vi "KM_appendline --readfreq.vi"(1 "freq":dbl format="%#_13g", 5 "append to file? (new file:F)":bool=TRUE, 7 "Save frequency scan":path=path "C:/data/Ultrasound/birdcage/Hg1201/Test", 8 "read/write control":T1, 9 "name or relative path":string) -> ()   [LabVIEW 2016]
uses:
  KM_file -- read-write control.ctl
  file -- read-write control.ctl
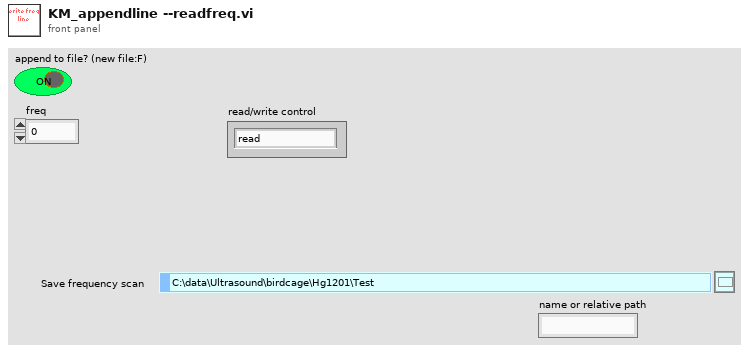
[diagram p1: front panel]
types:
  T1 = typedef "KM_file -- read-write control.ctl" = enum16{"read", "write all", "append one line"}
  T2 = typedef "file -- read-write control.ctl" = enum16{"read", "write all", "append one line"}
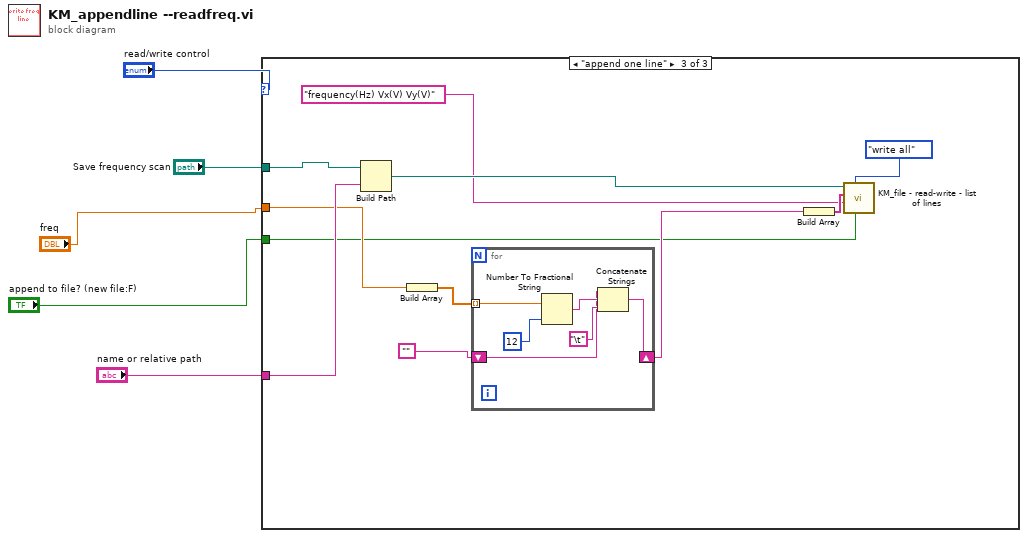
[diagram p0: block diagram]
diagram:
  n1 = case shown="\"append one line\"" "read/write control" {
    tunnel: "Save frequency scan" -> [_ _ w6]
    tunnel: "name or relative path" -> [_ _ w16]
    tunnel: "freq" -> [_ _ w9]
    tunnel: "append to file? (new file:F)" -> [_ _ w7]
    frame "read", Default {
    }
    frame "write all" {
    }
    frame "append one line" {
      n2 = Build Path(base path=w6, name or relative path=w16) -> (appended path=w11:path)
      n3 = Build Array(w9) -> (w15:dbl[])
      n4 = for {
        tunnel: w15 -> [w22] mode=indexing
        shift-right: [w18] -> w13
        shift-left: "" -> [w19]
        n5 = Number To Fractional String(number=w22, precision (6)=i16 12) -> (F-format string=w21:string)  [unwired: 2 in]
        n6 = Concatenate Strings(w19, w21, "\t" ("string")) -> (w18:string)
      }
      n7 = Build Array(w13) -> (w10:string[])
      n8 = call "KM_file - read-write - list of lines.vi"("append to file? (new file:F)"=w7, "read/write control"=file_--_read-write_control."write all", "header"="frequency(Hz) Vx(V) Vy(V)", "list of lines IN"=w10, "file path"=w11) -> ()  [unwired: 5 in, 2 out]
    }
  }
